vi "get param info.vi"(8 "错误输入（无错误）":errorcluster) -> (0 "错误输出":errorcluster, 3 "参数列表":string[][](array[string]))   [LabVIEW 2017]
uses:
  <userlib>/SimuLabAPIEx_V3/SimuLabAPIEx_V3.lvlib
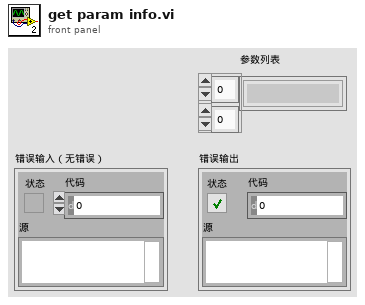
[diagram p1: front panel]
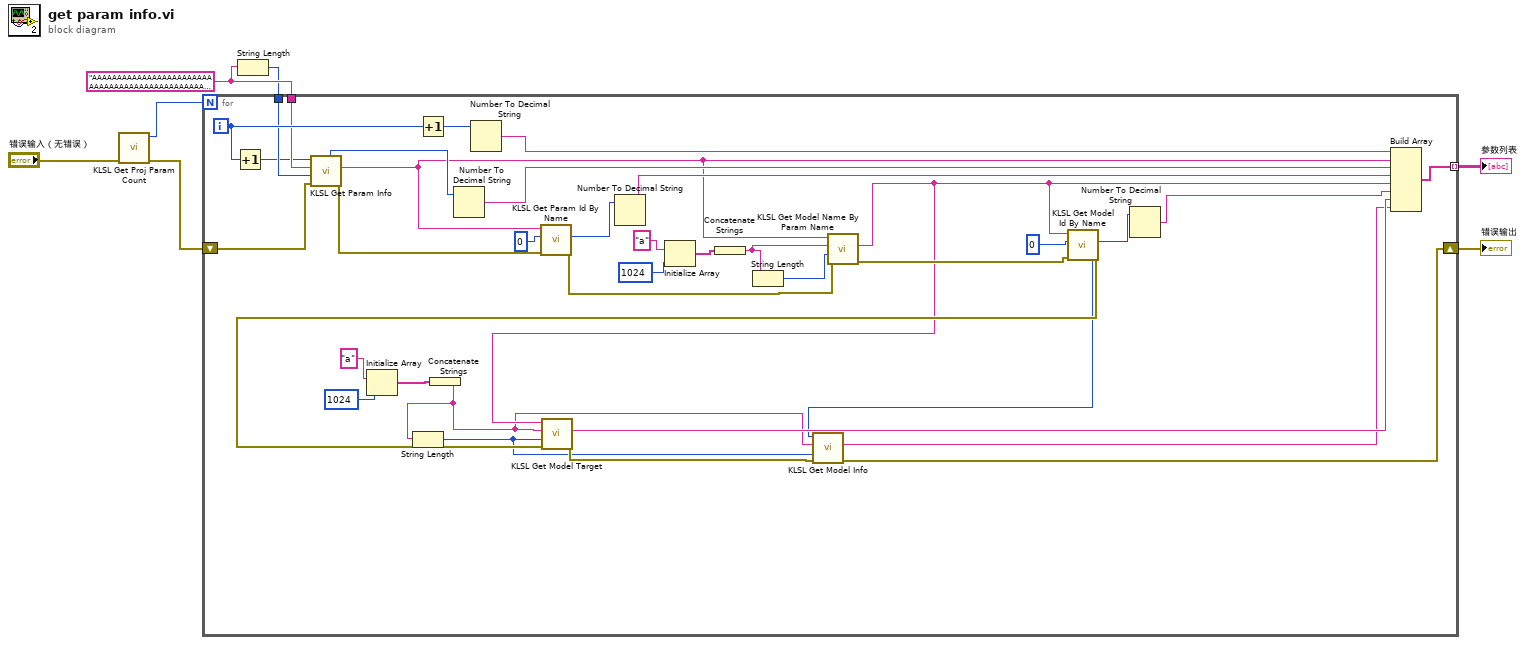
[diagram p0: block diagram]
diagram:
  w5 = "AAAAAAAAAAAAAAAAAAAAAAAAAAAAAAAAAAAAAAAAAAAAAAAAAAAAAAAAAAAAAAAAAAAAAAAAAAAAAAAAAAAAAAAAAAAAAAAAAAAAAAAAAAAAAAAAAAAAAAAAAAAAAAAAAAAAAAAAAAAAAAAAAAAAAAAAAAAAAAAAAAAAAAAAAAAAAAAAAAAAAAAAAAAAAAAAAAAAAAAAAAAAAAAAAAAAAAAAAAAAAAAAAAAAAAAAAAAAAAAAAAAAAAAAAAAAAAAA" ("szProjName")
  n1 = call <userlib>:"KLSL Get Proj Param Count.vi"("error in (no error)"="错误输入（无错误）") -> ("error out"=w2:errorcluster, "nCount out"=w1:i32)  [unwired: 8 in, 1 out]
  n2 = String Length(string=w5) -> (length=w4:i32)
  n3 = for {
    N: w1 -> [_]
    tunnel: w5 -> [w38]
    tunnel: w4 -> [w37]
    tunnel: [w40] -> w6 mode=indexing
    shift-right: [w12] -> w7
    shift-left: w2 -> [w36]
    i -> [w39]
    n4 = Increment(x=w39) -> (x+1=w34:i32)
    n5 = call <userlib>:"KLSL Get Param Info.vi"("error in (no error)"=w36, "nNameBuffLen"=w37, "szParamName"=w38, "nParamIndex"=w34) -> ("error out"=w33:errorcluster, "szParamName out"=w28:string, "nParamLength out"=w35:i32)  [unwired: 4 in, 1 out]
    n6 = Initialize Array("a", 1024) -> (w15:string[])
    n7 = Increment(x=w39) -> (x+1=w43:i32)
    n8 = Concatenate Strings(w15) -> (w10:string)
    n9 = String Length(string=w10) -> (length=w9:i32)
    n10 = Number To Decimal String(number=w35) -> (decimal integer string=w41:string)  [unwired: 1 in]
    n11 = Number To Decimal String(number=w43) -> (decimal integer string=w42:string)  [unwired: 1 in]
    n12 = call <userlib>:"KLSL Get Param Id By Name.vi"("error in (no error)"=w33, "nParamId"=0, "szParamName"=w28) -> ("error out"=w29:errorcluster, "nParamId out"=w31:i32)  [unwired: 6 in, 1 out]
    n13 = Number To Decimal String(number=w31) -> (decimal integer string=w30:string)  [unwired: 1 in]
    n14 = Initialize Array("a", 1024) -> (w25:string[])
    n15 = Concatenate Strings(w25) -> (w24:string)
    n16 = String Length(string=w24) -> (length=w23:i32)
    n17 = call <userlib>:"KLSL Get Model Name By Param Name.vi"("error in (no error)"=w29, "nNameBuffLen"=w23, "szModelName"=w24, "szParamName"=w28) -> ("error out"=w22:errorcluster, "szModelName out"=w18:string)  [unwired: 5 in, 1 out]
    n18 = call <userlib>:"KLSL Get Model Id By Name.vi"("error in (no error)"=w22, "nModelId"=0, "szModelName"=w18) -> ("error out"=w19:errorcluster, "nModelId out"=w11:i32)  [unwired: 6 in, 1 out]
    n19 = call <userlib>:"KLSL Get Model Target.vi"("error in (no error)"=w19, "nTargetBuffLen"=w9, "szTargetIp"=w10, "szModelName"=w18) -> ("error out"=w13:errorcluster, "szTargetIp out"=w14:string)  [unwired: 5 in, 1 out]
    n20 = call <userlib>:"KLSL Get Model Info.vi"("error in (no error)"=w13, "nNameBuffLen"=w9, "szModelName"=w10, "nModelIdx"=w11) -> ("error out"=w12:errorcluster, "szModelName out"=w8:string)  [unwired: 5 in, 1 out]
    n21 = Number To Decimal String(number=w11) -> (decimal integer string=w20:string)  [unwired: 1 in]
    n22 = Build Array(w42, w28, w41, w30, w18, w20, w14, w8) -> (w40:string[])
  }
  "参数列表" <- w6
  "错误输出" <- w7
